vi "Test DAQmx Lock-in.vi"() -> ()   [LabVIEW 2020]
uses:
  SoftwareLockin/Lock-in Detector/Lock-in Detector.lvclass
  SoftwareLockin/Lock-in Detector/Lock-in Detector.lvclass/Lock-in Detector.ctl
  <vilib>/DAQmx/read.llb/DAQmx Read (Analog 1D DBL 1Chan NSamp).vi
  SoftwareLockin/Lock-in Detector/Write Sample rate.vi
  SoftwareLockin/Lock-in Detector/Write Time constant.vi
  <vilib>/DAQmx/miscellaneous.llb/DAQmx Fill In Error Info.vi
  <vilib>/Analysis/2dsp.llb/Decimate (continuous, CDB).vi
  <resource>/objmgr/daqmx.rc
  <vilib>/Analysis/NI_AALPro.lvlib
panel:
  in  "Position scale":dbl=0.1 format="%#_6pV"
  out "Position":dbl(knob) scale=-90.0..90.0
  in  "Tab Control":enum32{"Main", "Diagnostics"}(tab)
  in  "Amplitude":dbl=0.04 format="%#_6pV"
  out "Angle":dbl
  out "R":dbl
  out "Y":dbl
  out "X":dbl
  out "Waveform Chart":dbl[](graph)
  in  "DAQmx Device Name":tag="Dev1"
  in  "Time constant":dbl=1.0 format="%#_6ps"
  in  "Frequency":dbl=96.0 format="%#_6pHz"
  in  "Stop Button":bool
  in  "Input channel":string="ai0"
  in  "Input range":dbl=1.0 format="%#_6pV"
  out "Waveform Graph":dbl[](graph)
  out "AvailSampPerChan":u32 format="%#_12p"
  out "Done":bool
  out "Done 2":bool
  out "error out":errorcluster
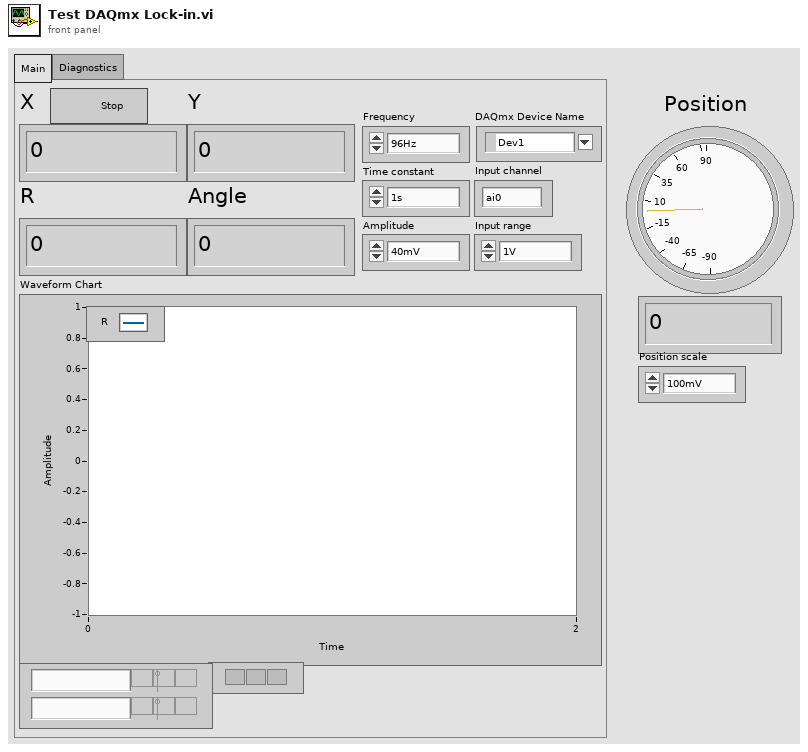
[diagram p1: front panel]
types:
  T1 = typedef "Lockin Parameters.ctl" = cluster{"Frequency":dbl, "Phase":dbl, "Syncronous":bool, "Points per sine wave":i32, "DDS":bool, "Frequency word":u32, "Phase word":u32, "DDS modulus":i64, "DDS clock":dbl}
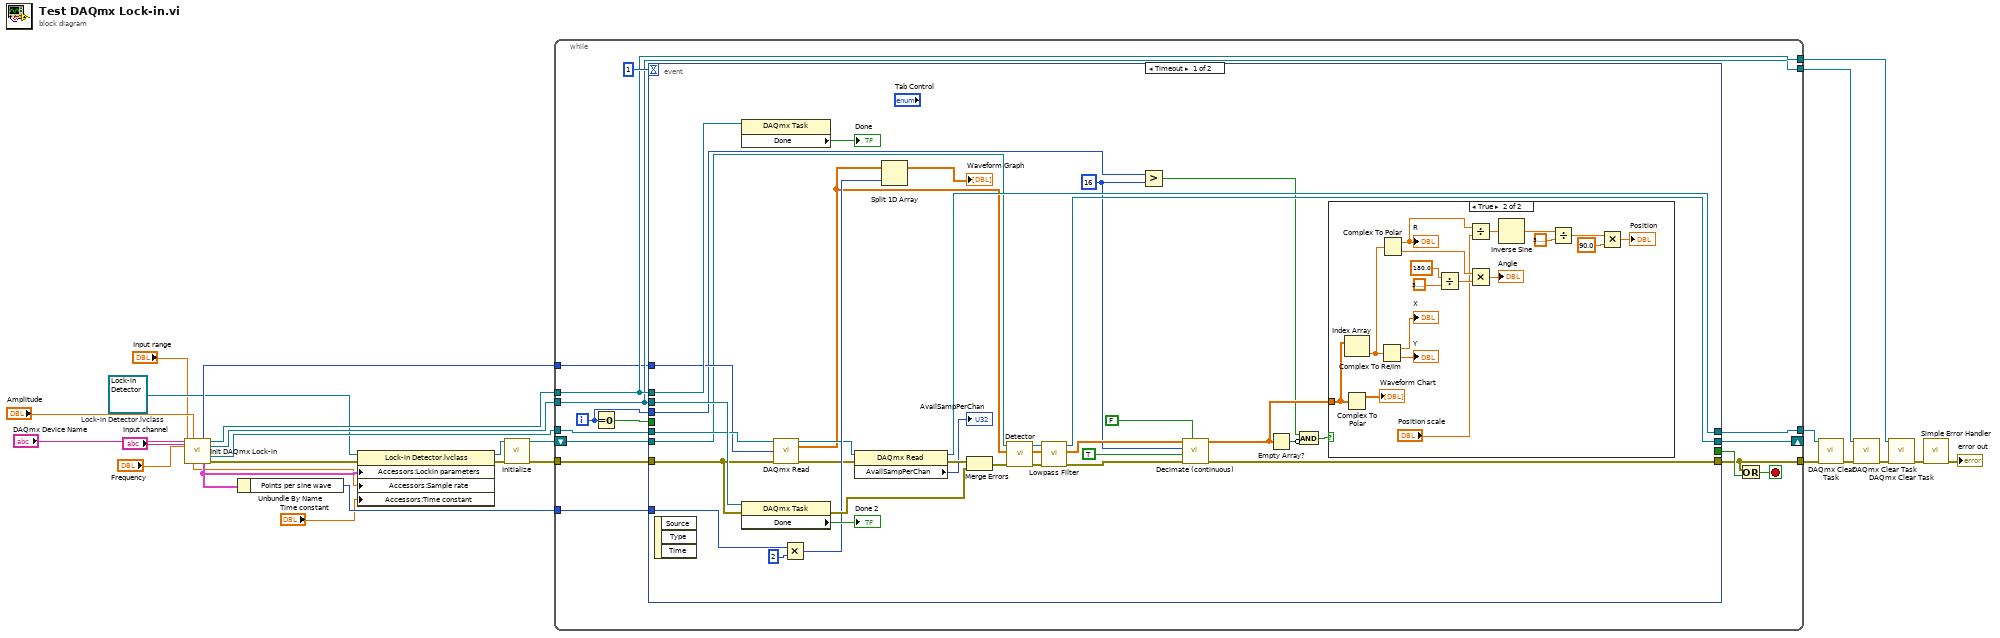
[diagram p0: block diagram]
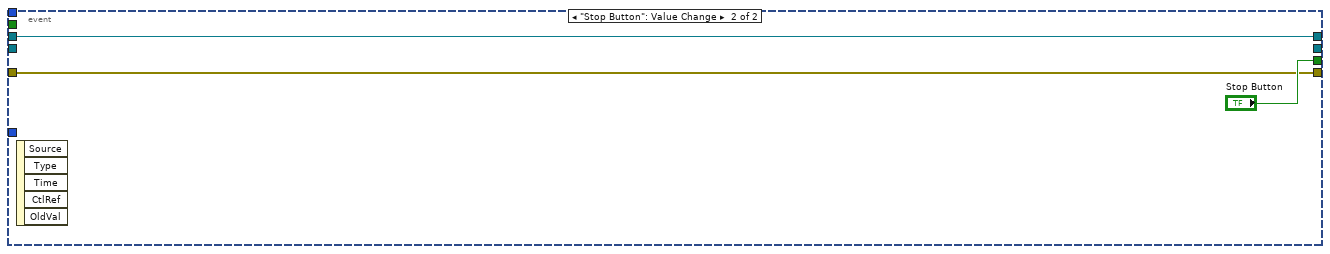
[diagram p3: hidden frame]
diagram:
  w13 = refnum<class "Lock-in Detector.lvclass"> refnum  # Lock-in Detector.lvclass
  n1 = call "Init DAQmx Lock-in.vi"("DAQmx Device Name"="DAQmx Device Name", "Amplitude"="Amplitude", "Desired frequency"="Frequency", "Input channel"="Input channel", "Input range"="Input range") -> ("Samples per read"=w14:i32, "CO task out"=w25:refnum<k21>, "AO task out"=w22:refnum<k21>, "AI task out"=w15:refnum<k21>, "Actual clock"=w8:dbl, "Lockin parameters"=w11:T1, "error out"=w5:errorcluster)  [unwired: 4 in]
  n2 = Unbundle By Name(w11) -> ("Points per sine wave"=w12:i32)
  n3 = property class="Lock-in Detector.lvclass"(reference=w13, error in=w5, "Accessors:Lockin parameters"=w11, "Accessors:Sample rate"=w8, "Accessors:Time constant"="Time constant") -> (reference out=w10:refnum<class "Lock-in Detector.lvclass">, error out=w9:errorcluster)
  n4 = call-dynamic "Initialize.vi"("error in (no error)"=w9, "Software Lock-in in"=w10) -> ("error out"=w6:errorcluster, "Software Lock-in out"=w7:refnum<class "Lock-in Detector.lvclass">)  [unwired: 7 in, 1 out]
  n5 = while {
    tunnel: w25 -> [w40]
    tunnel: [w40] -> w24
    tunnel: [w39] -> w23
    tunnel: w22 -> [w39]
    tunnel: w6 -> [w36]
    tunnel: [w37] -> w18
    tunnel: [w35] -> w16
    tunnel: w15 -> [w34]
    tunnel: w14 -> [w33]
    tunnel: w12 -> [w32]
    shift-right: [w30] -> _
    shift-left: w7 -> [w31]
    i -> [w28]
    stop <- w38 stop-if-true
    n6 = Equal To 0?(x=w28) -> (x = 0?=w29:bool)
    n7 = event shown="[0] Timeout" {
      selector: _ -> [_ _]
      dyn-events: _ -> [_ _]
      timeout: 1 -> [_ _]
      tunnel: [_ "Stop Button"] -> w42
      tunnel: w40 -> [w77 _]
      tunnel: w39 -> [w75 _]
      tunnel: [w51 w96] -> w37
      tunnel: w36 -> [w71 w96]
      tunnel: w34 -> [w72 w97]
      tunnel: [w62 w97] -> w35
      tunnel: w33 -> [w70 _]
      tunnel: w32 -> [w69 _]
      tunnel: w31 -> [w60 _]
      tunnel: [w58 _] -> w30
      tunnel: w29 -> [_ _]
      tunnel: w28 -> [w47 _]
      event Timeout {
        w45 = 16 ("decimating factor")
        n8 = event-data() -> ()  [unwired: 1 in, 3 out]
        n9 = property class="DAQmx Task"(reference=w77) -> ("Done"=→"Done":bool)  [unwired: 1 in, 2 out]
        n10 = property class="DAQmx Task"(reference=w75, error in=w71) -> (error out=w73:errorcluster, "Done"=→"Done 2":bool)  [unwired: 1 out]
        n11 = call-poly <vilib>:"DAQmx Read.vi"("task/channels in"=w72, "number of samples per channel"=w70, "error in"=w71) -> ("task out"=w65:refnum<k21>, "data"=w55:dbl[], "error out"=w64:errorcluster)  [unwired: 10 in]
        n12 = Multiply(x=w69, y=2) -> (x*y=w68:i32)
        n13 = property class="DAQmx Read"(reference=w65, error in=w64) -> (reference out=w62:refnum<k21>, error out=w63:errorcluster, "AvailSampPerChan"=→"AvailSampPerChan":u32)
        n14 = Split 1D Array(array=w55, index=w68) -> (first subarray=→"Waveform Graph":dbl[])  [unwired: 1 out]
        n15 = Merge Errors(w63, w73) -> (w56:errorcluster)
        n16 = call-dynamic "Detector.vi"("error in (no error)"=w56, "Signal"=w55, "Lock-in Detector in"=w60) -> ("error out"=w57:errorcluster, "Signal out"=w54:cdb[], "Lock-in Detector out"=w59:refnum<class "Lock-in Detector.lvclass">)  [unwired: 6 in]
        n17 = call-dynamic "Lowpass Filter.vi"("error in (no error)"=w57, "Signal"=w54, "Lock-in Detector in"=w59) -> ("error out"=w53:errorcluster, "Signal out"=w50:cdb[], "Lock-in Detector out"=w58:refnum<class "Lock-in Detector.lvclass">)  [unwired: 6 in]
        n18 = Greater?(x=w47, y=w45) -> (0:w46:bool)
        n19 = call-poly <vilib>:"Decimate (continuous).vi"("reset"=FALSE, "error in (no error)"=w53, "averaging"=TRUE, "decimating factor"=w45, "X"=w50) -> ("error out"=w51:errorcluster, "Decimated Array"=w49:cdb[])  [unwired: 5 in]
        n20 = Empty Array?(array=w49) -> (empty?=w43:bool)
        n21 = Compound Arithmetic op=AND(w46, invert w43) -> (w44:bool)
        n22 = case shown="True" w44 {
          tunnel: w49 -> [_ w94]
          frame False {
          }
          frame True {
            n23 = Index Array(array=w94) -> (element=w92:cdb)  [unwired: 1 in]
            n24 = Complex To Polar(r * e^(i*theta)=w94) -> (r=→"Waveform Chart":dbl[])  [unwired: 1 out]
            n25 = Complex To Re/Im(x + iy=w92) -> (x=→"X":dbl, y=→"Y":dbl)
            n26 = Complex To Polar(r * e^(i*theta)=w92) -> (r=w85:dbl, theta=w93:dbl)
            "R" <- w85
            n27 = Divide(x=180.0, y=3.141592653589793) -> (x/y=w87:dbl)
            n28 = Divide(x=w85, y="Position scale") -> (x/y=w83:dbl)
            n29 = Multiply(x=w93, y=w87) -> (x*y=→"Angle":dbl)
            n30 = Inverse Sine(1:w83) -> (0:w82:dbl)
            n31 = Divide(x=w82, y=3.141592653589793) -> (x/y=w80:dbl)
            n32 = Multiply(x=w80, y=90.0) -> (x*y=→"Position":dbl)
          }
        }
      }
      event "Stop Button": Value Change {
        n33 = event-data() -> ()  [unwired: 1 in, 5 out]
      }
    }
    n34 = Or(x=w37, y=w42) -> (x .or. y?=w38:bool)
  }
  n35 = call <vilib>:"DAQmx Clear Task.vi"("task in"=w16, "error in"=w18) -> ("error out"=w17:errorcluster)  [unwired: 13 in]
  n36 = call <vilib>:"DAQmx Clear Task.vi"("task in"=w23, "error in"=w17) -> ("error out"=w20:errorcluster)  [unwired: 13 in]
  n37 = call <vilib>:"DAQmx Clear Task.vi"("task in"=w24, "error in"=w20) -> ("error out"=w19:errorcluster)  [unwired: 13 in]
  n38 = call <vilib>:"Simple Error Handler.vi"("error in (no error)"=w19) -> ("error out"=→"error out":errorcluster)  [unwired: 4 in, 4 out]
